vi "ProdLimits.vi"(8 "error in (no error)":errorcluster, 11 "*.ini file":path=path "C:/3500004_TetraProductionReportGenerator/testreport.ini") -> (0 "error out":errorcluster, 2 "Prod_limits":cluster{"names":string, "limits":dbl}[](array[cluster]))   [LabVIEW 2018]
uses:
  <vilib>/Utility/error.llb/Error Cluster From Error Code.vi
  Tetra_Globals.vi
  <vilib>/ErrorRing/Error Ring.xnode
panel:
  out "ok?":bool
  out "standalone(t)":bool
  out "file text":string
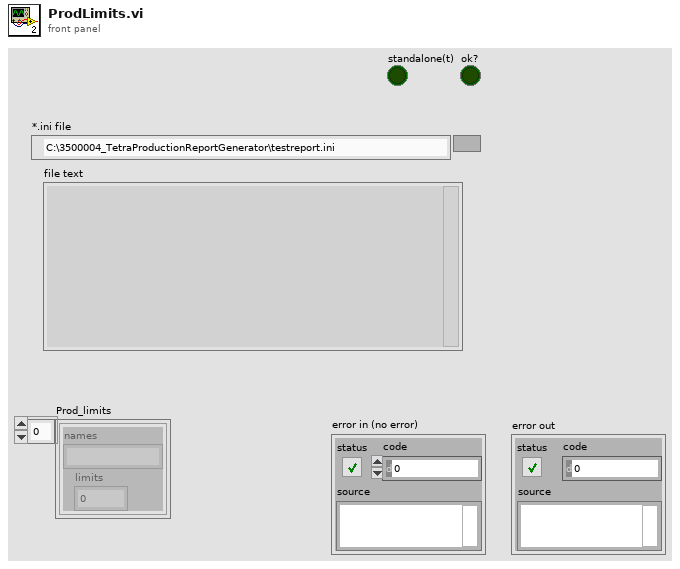
[diagram p1: front panel]
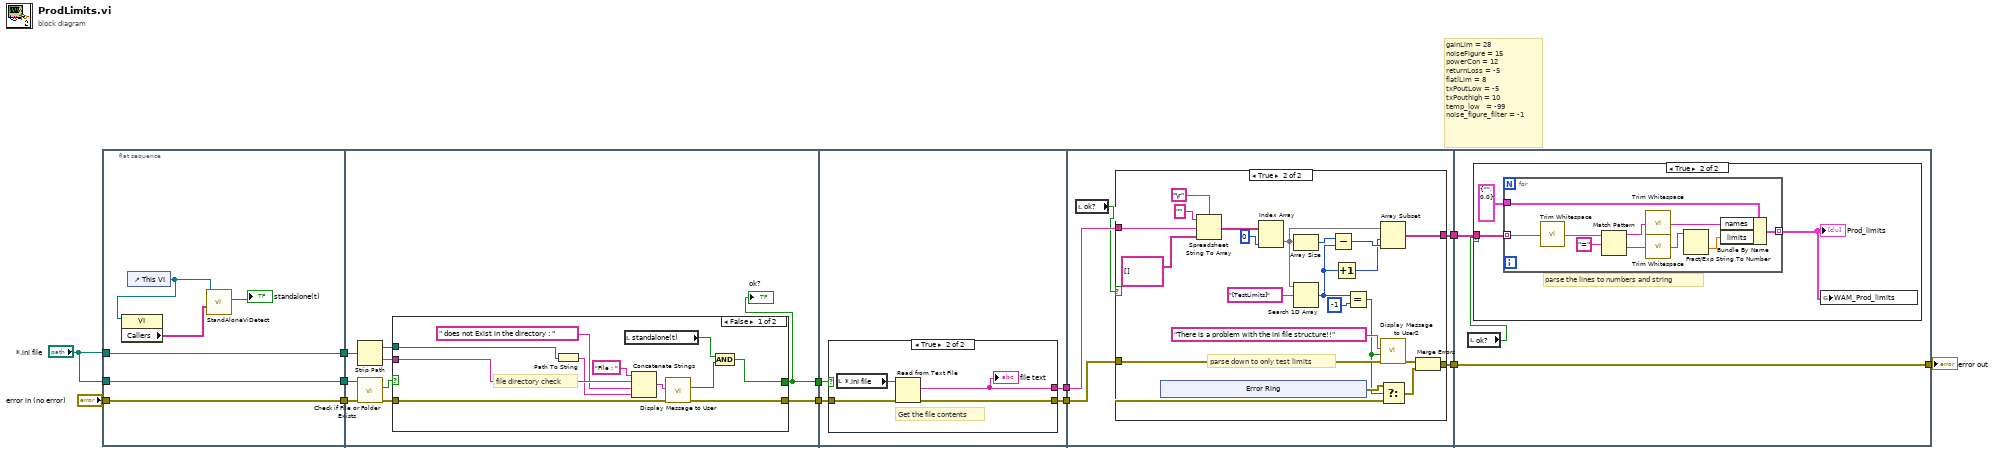
[diagram p0: block diagram]
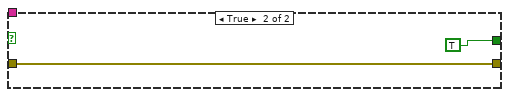
[diagram p2: hidden frame]
diagram:
  # "gainLim = 28\nnoiseFigure = 15\npowerCon = 12\nreturnLoss = -5\nflatlLim = 8\ntxPoutLow = -5\ntxPouthigh = 10\ntemp_low   = -99\nnoise_figure_filter = -1"
  n1 = flat-sequence {
    tunnel: "*.ini file" -> [w16]
    tunnel: "error in (no error)" -> [w17]
    tunnel: "*.ini file" -> [w18]
    tunnel: [w18] -> w4
    tunnel: [w17] -> w3
    tunnel: [w16] -> w2
    tunnel: [w25] -> w9
    tunnel: w4 -> [w22]
    tunnel: w3 -> [w23]
    tunnel: w2 -> [w27]
    tunnel: [w19] -> w1
    tunnel: [w44] -> w12
    tunnel: w9 -> [w43]
    tunnel: [w42] -> w8
    tunnel: w1 -> [w41]
    tunnel: w12 -> [w54]
    tunnel: w8 -> [w52]
    tunnel: [w53] -> w6
    tunnel: [w51] -> w5
    tunnel: [w84] -> w7
    tunnel: w6 -> [w84]
    tunnel: w5 -> [w83]
    frame #0 {
      n2 = control-ref of="This VI"() -> (w15:refnum<vi>)
      n3 = property class="VI"(reference=w15) -> ("Callers"=w14:string[])  [unwired: 1 in, 2 out]
      n4 = call "StandAloneViDetect.vi"("call chain"=w14, "VI in"=w15) -> ("standalone(t)"=→"standalone(t)":bool)  [unwired: 8 in, 1 out]
    }
    frame #1 {
      n5 = Strip Path(path=w22) -> (stripped path=w21:path, name=w20:string)
      n6 = call <vilib>:"Check if File or Folder Exists.vi"("error in (no error)"=w23, "path"=w27) -> ("error out"=w24:errorcluster, "file or folder exists?"=w26:bool)  [unwired: 7 in, 1 out]
      n7 = case shown="False" w26 {
        tunnel: w24 -> [w37 w40]
        tunnel: [w38 w40] -> w25
        tunnel: w21 -> [w33 _]
        tunnel: w20 -> [w36 _]
        tunnel: [w28 TRUE] -> w19
        frame False {
          # "file directory check"
          n8 = Path To String(path=w33) -> (string=w32:string)
          n9 = local read "standalone(t)"() -> (w29:bool)
          n10 = Concatenate Strings("File : " ("string"), w36, " does not Exist in the directory : " ("string"), w32) -> (w31:string)
          n11 = call "Display Message to User"("error in (no error)"=w37, "Message"=w31) -> ("error out"=w38:errorcluster, "OK"=w30:bool)  [unwired: 8 in]
          n12 = And(x=w29, y=w30) -> (x .and. y?=w28:bool)
        }
        frame True {
        }
      }
      "ok?" <- w19
    }
    frame #2 {
      n13 = case shown="True" w41 {
        tunnel: [_ w49] -> w44
        tunnel: w43 -> [w45 w48]
        tunnel: [w45 w46] -> w42
        frame False {
        }
        frame True {
          # "Get the file contents"
          n14 = local read "*.ini file"() -> (w47:path)
          n15 = Read from Text File(file (use dialog)=w47, error in=w48) -> (text=w49:string, error out=w46:errorcluster)  [unwired: 2 in, 2 out]
          "file text" <- w49
        }
      }
    }
    frame #3 {
      n16 = local read "ok?"() -> (w50:bool)
      n17 = case shown="True" w50 {
        tunnel: w54 -> [_ w67]
        tunnel: [w55 w61] -> w53
        tunnel: w52 -> [w55 w58]
        tunnel: [_ w57] -> w51
        frame False {
        }
        frame True {
          # "parse down to only test limits"
          n18 = xnode "Error Ring"() -> ("error out"=w59:errorcluster)
          n19 = Spreadsheet String To Array(delimiter (Tab)="\r", format string="", spreadsheet string=w67, array type (2D Dbl)=string[][] []) -> (array=w65:string[][])
          n20 = Index Array(array=w65, index (col)=0 ("disabled index (col)")) -> (element=w70:string[])  [unwired: 1 in]
          n21 = Array Size(array=w70) -> (size(s)=w74:i32)
          n22 = Search 1D Array(1D array=w70, element="[TestLimits]" ("regular expression")) -> (index of element=w73:i32)  [unwired: 1 in]
          n23 = Subtract(x=w74, y=w73) -> (x-y=w72:i32)
          n24 = Increment(x=w73) -> (x+1=w64:i32)
          n25 = Equal?(x=w73, y=-1) -> (x = y?=w56:bool)
          n26 = Array Subset(array=w70, index=w64, length=w72) -> (w57:string[])
          n27 = call "Display Message to User2"("error in (no error)"=w58, "Enable"=w56, "Message"="There is a problem with the ini file structure!!") -> ("error out"=w63:errorcluster)  [unwired: 7 in, 1 out]
          n28 = Select(t=w59, s=w56, f=w58) -> (s? t:f=w60:errorcluster)
          n29 = Merge Errors(w63, w60) -> (w61:errorcluster)
        }
      }
    }
    frame #4 {
      n30 = local read "ok?"() -> (w82:bool)
      n31 = case shown="True" w82 {
        tunnel: w83 -> [_ w87]
        frame False {
        }
        frame True {
          # "parse the lines to numbers and string"
          n32 = for {
            tunnel: w87 -> [w97] mode=indexing
            tunnel: [w89] -> w85 mode=indexing
            tunnel: cluster{"names":string, "limits":dbl} {"names"="", "limits"=0.0} ("output cluster") -> [w88]
            n33 = call <vilib>:"Trim Whitespace.vi"("string"=w97) -> ("trimmed string"=w95:string)  [unwired: 1 in]
            n34 = Match Pattern(string=w95, regular expression="=") -> (before substring=w92:string, after substring=w94:string)  [unwired: 1 in, 2 out]
            n35 = call <vilib>:"Trim Whitespace.vi"("string"=w92) -> ("trimmed string"=w91:string)  [unwired: 1 in]
            n36 = call <vilib>:"Trim Whitespace.vi"("string"=w94) -> ("trimmed string"=w93:string)  [unwired: 1 in]
            n37 = Fract/Exp String To Number(string=w93) -> (number=w90:dbl)  [unwired: 3 in, 1 out]
            n38 = Bundle By Name(cluster=w88, "names"=w91, "limits"=w90) -> (w89:cluster{"names":string, "limits":dbl})
          }
          "Prod_limits" <- w85
          n39 = global write "Tetra_Globals.vi" "WAM_Prod_limits"(w85) -> ()
        }
      }
    }
  }
  "error out" <- w7
